vi "NDMotor_TransToSteps.vi"(11 "Transmission":i32) -> (3 "Steps":i32)   [LabVIEW 2024]
uses:
  <vilib>/Analysis/polynomials.llb/Scalar Polynomial Evaluation (DBL).vi
  <vilib>/Analysis/polynomials.llb/1D Polynomial Evaluation (DBL).vi
  <vilib>/Analysis/NI_AALPro.lvlib
panel:
  out "XY Graph":cluster{dbl[], "P(A)":dbl[]}(graph)
  in  "Step":dbl=0.1 format="%_6g"
  in  "Final":dbl=5.4 format="%_6g"
  in  "Initial":dbl=0.7 format="%_6g"
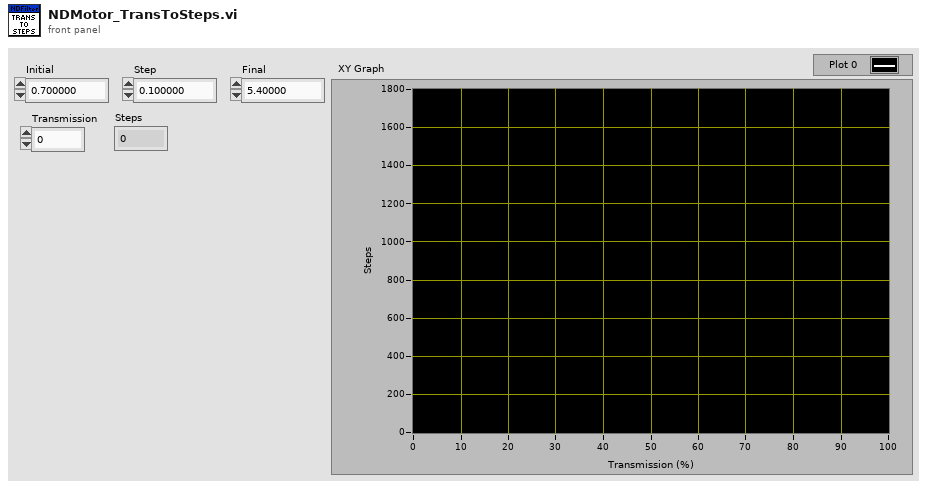
[diagram p1: front panel]
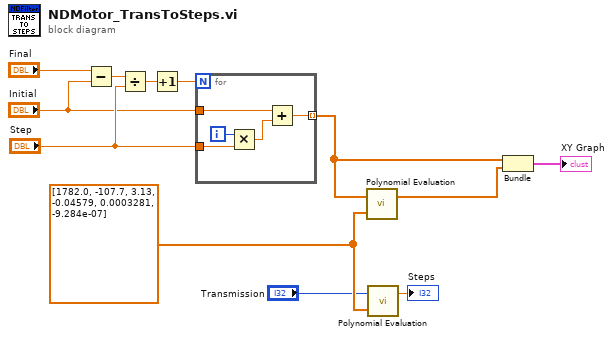
[diagram p0: block diagram]
diagram:
  w8 = dbl[] [1782.0, -107.7, 3.13, -0.04579, 0.0003281, -9.284e-07] ("P(x)")
  n1 = Subtract(x="Final", y="Initial") -> (x-y=w12:dbl)
  n2 = Divide(x=w12, y="Step") -> (x/y=w10:dbl)
  n3 = Increment(x=w10) -> (x+1=w9:dbl)
  n4 = for {
    N: w9 -> [_]
    tunnel: "Step" -> [w16]
    tunnel: "Initial" -> [w15]
    tunnel: [w13] -> w2 mode=indexing
    i -> [w17]
    n5 = Multiply(x=w17, y=w16) -> (x*y=w14:dbl)
    n6 = Add(x=w15, y=w14) -> (x+y=w13:dbl)
  }
  n7 = call-poly <vilib>:"Polynomial Evaluation.vi"("P(x)"=w8, "A"=w2) -> ("P(A)"=w1:dbl[])  [unwired: 1 out]
  n8 = call-poly <vilib>:"Polynomial Evaluation.vi"("P(x)"=w8, "a"="Transmission") -> ("P(a)"=→"Steps":dbl)  [unwired: 1 out]
  n9 = Bundle(w2, "P(A)"=w1) -> (→"XY Graph":cluster{dbl[], "P(A)":dbl[]})  [unwired: 1 in]
